vi "Vsg from folder.vi"(11 "path":path) -> (3 "Numeric":dbl)   [LabVIEW 2016]
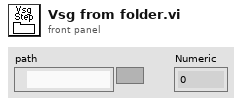
[diagram p1: front panel]
types:
  T1 = typedef "File Info Record__ogtk.ctl" = cluster{"type":string, "creator":string, "permissions":i32, "data size":i32, "res size":i32, "creation date":u32, "modification date":u32, "bFolder":bool, "bInvisible":bool, "location":cluster{"vertical":i16, "horizontal":i16}, "owner":string, "group":string}
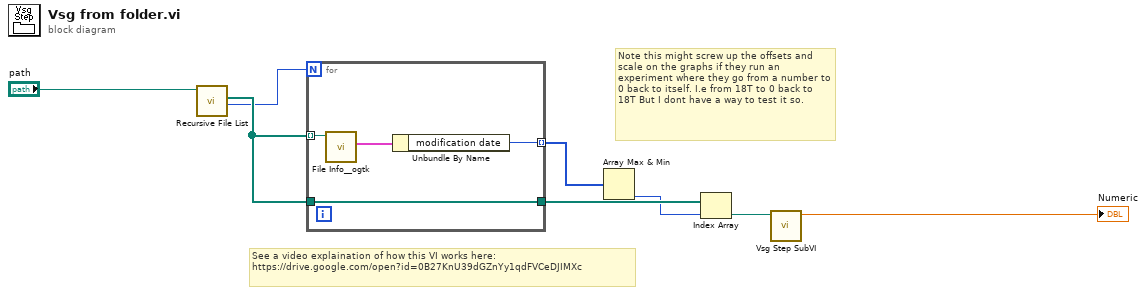
[diagram p0: block diagram]
diagram:
  # "Note this might screw up the offsets and scale on the graphs if they run an experiment where they go from a number to 0 back to itself. I.e from 18T to 0 back to 18T But I dont have a way to test it so."
  # "See a video explaination of how this VI works here: \nhttps://drive.google.com/open?id=0B27KnU39dGZnYy1qdFVCeDJIMXc"
  n1 = call <vilib>:"Recursive File List.vi"("Folder Path"="path") -> ("Number of Files"=w1:i32, "All Files in Dir"=w6:path[])  [unwired: 7 in, 2 out]
  n2 = for {
    N: w1 -> [_]
    tunnel: w6 -> [w11] mode=indexing
    tunnel: [w10] -> w3 mode=indexing
    tunnel: [w9] -> w5
    tunnel: w6 -> [w9]
    n3 = call <userlib>:"File Info__ogtk.vi"("file"=w11) -> ("file info"=w12:T1)  [unwired: 5 in, 2 out]
    n4 = Unbundle By Name(w12) -> ("modification date"=w10:u32)
  }
  n5 = Array Max & Min(array=w3) -> (min index (indices)=w2:i32)  [unwired: 3 out]
  n6 = Index Array(array=w5, index=w2) -> (element=w7:path)
  n7 = call "Vsg Step SubVI.vi"("file (use dialog) in"=w7) -> ("Numeric"=→"Numeric":dbl)  [unwired: 10 in]
